vi "Production to internal EEPROM.vi"(8 "error in":errorcluster) -> (0 "error out":errorcluster, 1 "Report":string, 2 "Pass?":bool, 3 "VISA Port":refnum<visa-resource-name>, 5 "DataTime":string, 7 "BOOTVER":string, 10 "BOOTVER":bool, 11 "Time&date":bool)   [LabVIEW 2009]
uses:
  Digit IO PCI 6503/Digit IO control.ctl
  Global/Global 1.vi
  <vilib>/Instr/_visa.llb/VISA Configure Serial Port (Instr).vi
panel:
  out "Path":path=path "E:/LCU6331 test/4821683A000/Config/configration file/Limits_Production.txt"
  out "Interal EEPROM":string
  out "APPVER":bool
  out "APPVER":string
  out "time":timestamp
  out "VerifyTime":string
  out "command Prob2":string
  out "command Prob1":string
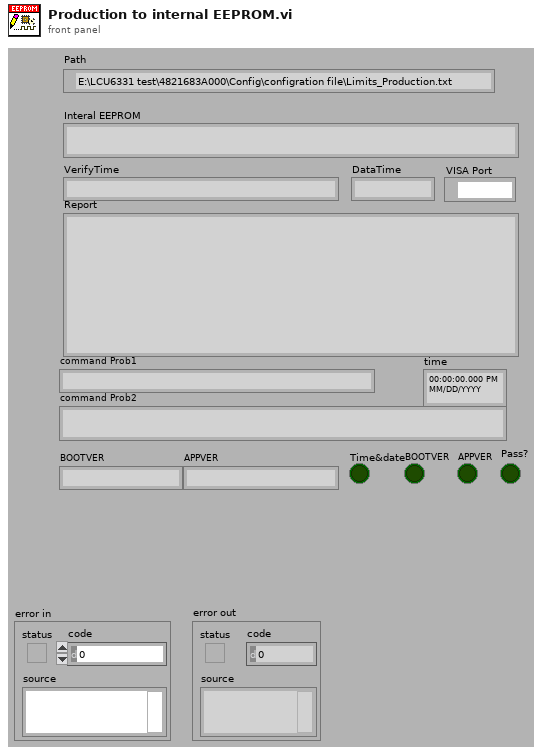
[diagram p1: front panel]
types:
  T1 = typedef "Digit IO control.ctl" = enum16{"Pull X1_4 Low", "Disconnect Pull X1_4 Low", "Down Cylinder", "Disconnect Down Cylinder", "Load X1_1_5", "Disconnect Load X1_1_5", "Measu X1_1_5", "Disconnect Measu X1_1_5", "Measu Z1_1_5", "Disconnect Measu Z1_1_5", "Power X1_1", "Disconnect Power X1_1", "RS232 Power", "Disconnect RS232 Power", "Card Cylinder", "Disconnect Card Cylinder", "Fail LED", "Disconnect Fail LED", "LCA Power", "Disconnect LCA Power", "BeyondCylinderDowndigit", "Disconnect BeyondCylinderDowendigit", "Frequency", "Disconnect Frequency", "Measu Current", "Disconnect Measu Current", "Measu current_1", "Disconnect Measu current_1", "Digit ALL", "Disconnect Digit ALL", "PASS LED", "Disconnect PASS LED", "Load Z1_1_3", "Disconnect Load Z1_1_3", "RS232 Connect", "Disconnect RS232 Connect", "Power Z1_7", "Disconnect Power Z1_7", "Pull Z_1_5  low", "Disconnect Pull Z_1_5  low", "Connect LCA_1", "Disconnect LCA_1", "short LCA", "Disconnect short LCA", "PT100", "Disconnect PT100", "NO connect", "Disconnect NO connect"}
  T2 = enum16{"VHEATFUSENOLOADMIN", "VHEATFUSELOADMAX", "VOVERRIDEDIODEMIN", "TDIFFMAX", "MEASFREQMIN", "MEASFREQMAX", "VMIDDLE", "VUNDER", "VNORESET", "VRESET", "WAITPING", "LRFID", "RFIDUID", "EXTEESIZE", "LCUTYPE", "LCUSUBTYPE", "TEVN", "BOOTVER", "APPVER", "ISLEEPMAX", "TSLEEP", "APPWAIT", "DBWAIT"}[]
  T3 = enum16{"LCU Power on", "Calculating time and date", "Command _E & DATA", "Command_E & String", "Read&Verify data", "Finish"}
  T4 = cluster{"People":string, "product  number":string, "Test time":string, "VHeatFuse_noload":string, "VHeatFuse_load":string, "VoverrideDiode":string, "Test firmware upload via X1":string, "TemperAddress":string, "Troom":string, "TLCU":string, "Adjustment factor":string, "MeasuredFreq":string, "I2C communication":string, "Light-emitting diode on Z2":string, "Battery warning/inhibit":string, "Reset by IC10":string, "External EEPROM":string, "RFID card detection and reading RFID":string, "Production parameters in internal EEPROM":string, "Current consumption in sleep mode":string, "Application and database upload":string, "Test result":string, "Table head[22]":string, "Table head[23]":string}
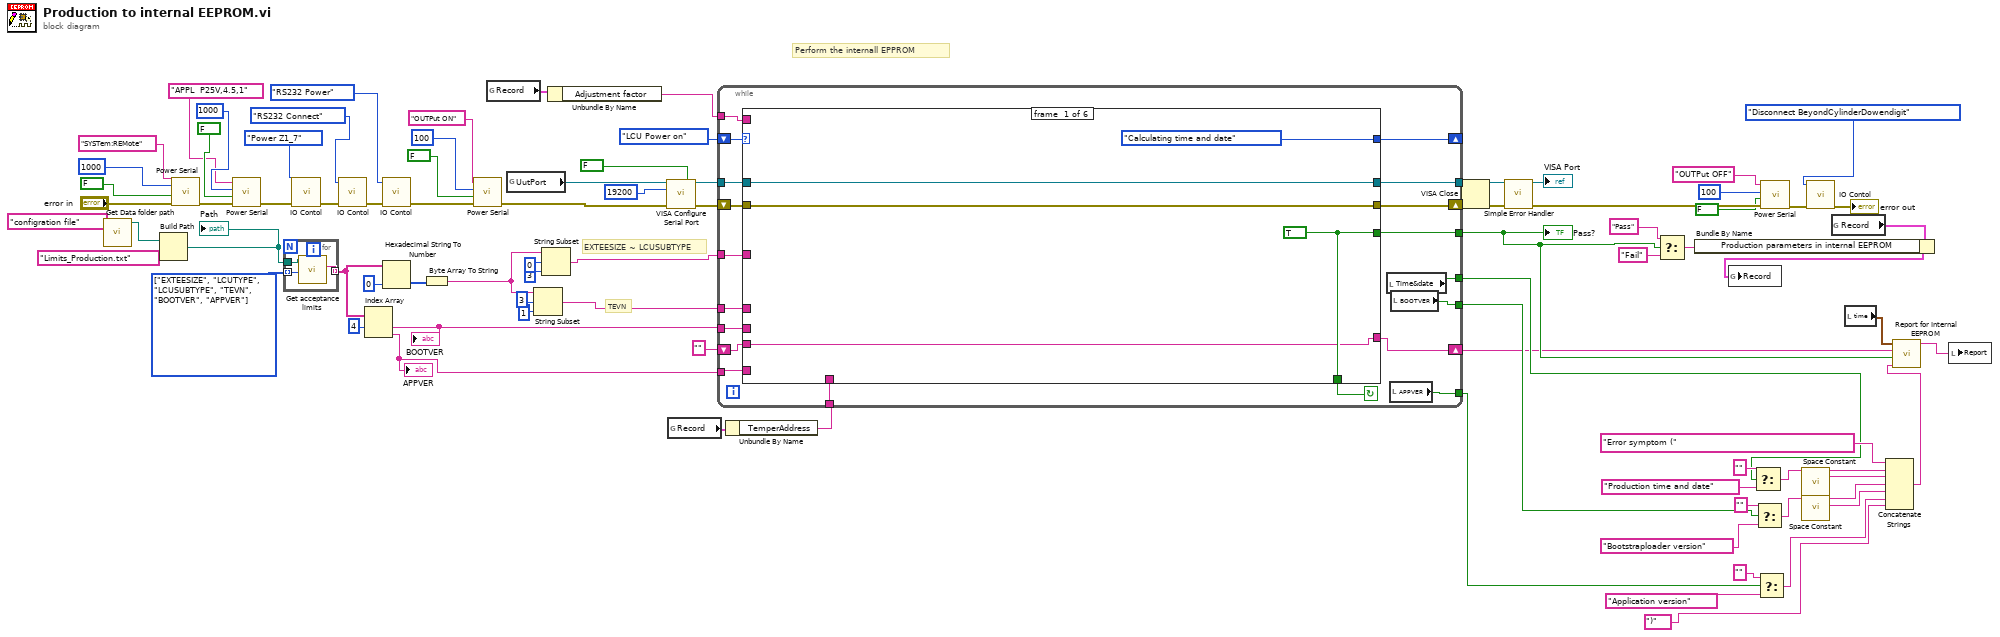
[diagram p0: block diagram]
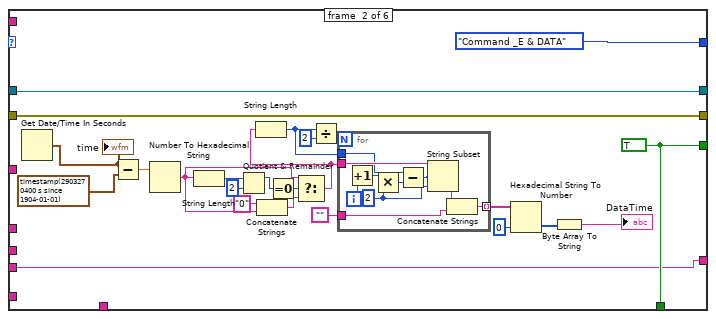
[diagram p2: hidden frame]
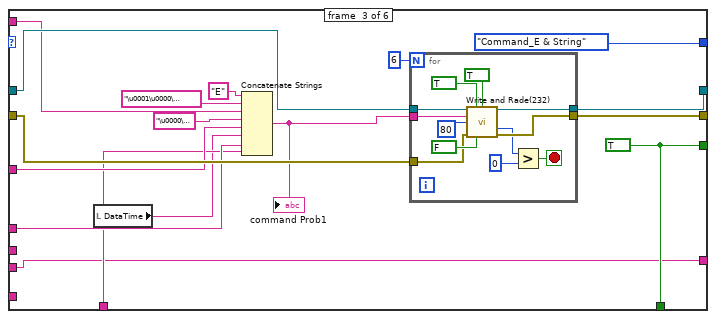
[diagram p3: hidden frame]
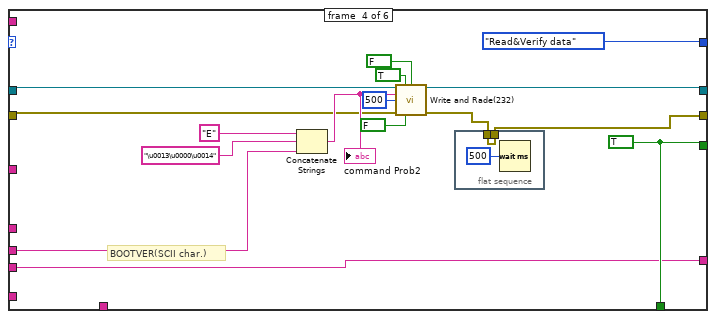
[diagram p4: hidden frame]
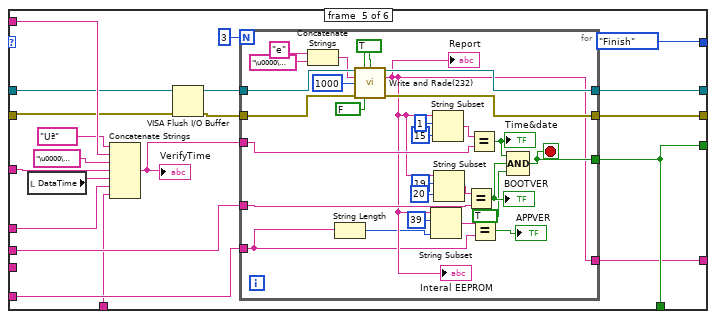
[diagram p5: hidden frame]
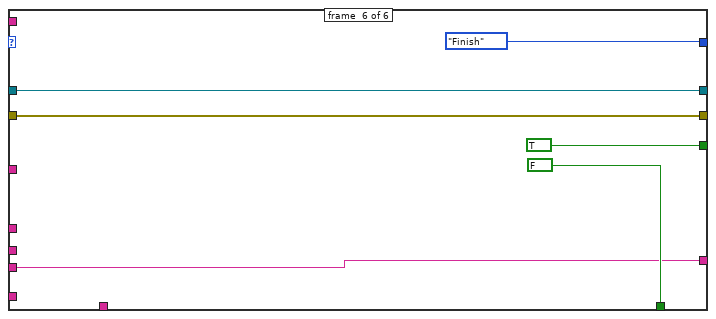
[diagram p6: hidden frame]
diagram:
  w71 = T2 [enum."EXTEESIZE", enum."LCUTYPE", enum."LCUSUBTYPE", enum."TEVN", enum."BOOTVER", enum."APPVER"] items=["VHEATFUSENOLOADMIN", "VHEATFUSELOADMAX", "VOVERRIDEDIODEMIN", "TDIFFMAX", "MEASFREQMIN", "MEASFREQMAX", "VMIDDLE", "VUNDER", "VNORESET", "VRESET", "WAITPING", "LRFID", "RFIDUID", "EXTEESIZE", "LCUTYPE", "LCUSUBTYPE", "TEVN", "BOOTVER", "APPVER", "ISLEEPMAX", "TSLEEP", "APPWAIT", "DBWAIT"]
  # "EXTEESIZE ~ LCUSUBTYPE"
  # "TEVN"
  # "Perform the internall EPPROM"
  n1 = call "Get Data folder path.vi"("Data Path Name"="configration file") -> ("Data Path"=w2:path)  [unwired: 1 in, 9 out]
  n2 = Build Path(base path=w2, name or relative path="Limits_Production.txt") -> (appended path=w1:path)
  "Path" <- w1
  n3 = call "Power Serial.vi"("error in (no error)"="error in", "Rd?"=FALSE, "Delay"=1000, "IN"="SYSTem:REMote" ("In")) -> ("error out"=w53:errorcluster)  [unwired: 1 in, 6 out]
  n4 = call "Power Serial.vi"("error in (no error)"=w53, "Rd?"=FALSE, "Delay"=1000, "IN"="APPL  P25V,4.5,1" ("In")) -> ("error out"=w40:errorcluster)  [unwired: 1 in, 6 out]
  n5 = for {
    tunnel: w1 -> [w87]
    tunnel: [w86] -> w6 mode=indexing
    tunnel: w71 -> [w85] mode=indexing
    n6 = call "Get acceptance limits.vi"("section"=w85, "configuration file path"=w87) -> ("value"=w86:string)  [unwired: 1 in, 8 out]
  }
  n7 = call "IO Contol.vi"("error in"=w40, "IO Operation"=Digit_IO_control."Power Z1_7" ("Enum")) -> ("error out"=w44:errorcluster)  [unwired: 9 out]
  n8 = call "IO Contol.vi"("error in"=w44, "IO Operation"=Digit_IO_control."RS232 Connect" ("Enum")) -> ("error out"=w45:errorcluster)  [unwired: 9 out]
  n9 = Index Array "Index Array"(array=w6, index #1=4 ("index")) -> (element #1=w10:string, element #2=w12:string)  [unwired: 1 in]
  "APPVER" <- w12
  "BOOTVER" <- w10
  n10 = call "IO Contol.vi"("error in"=w45, "IO Operation"=Digit_IO_control."RS232 Power" ("Enum")) -> ("error out"=w36:errorcluster)  [unwired: 9 out]
  n11 = Hexadecimal String To Number(string=w6, default (0uL)=u8 0) -> (number=w5:u8[])  [unwired: 2 out]
  n12 = Byte Array To String(unsigned byte array=w5) -> (string=w66:string)
  n13 = call "Power Serial.vi"("error in (no error)"=w36, "Rd?"=FALSE, "Delay"=100, "IN"="OUTPut ON" ("In")) -> ("error out"=w62:errorcluster)  [unwired: 1 in, 6 out]
  n14 = global read "Global 1.vi" "Record"() -> (w32:T4)
  n15 = global read "Global 1.vi" "UutPort"() -> (w61:refnum<visa-resource-name>)
  n16 = String Subset(string=w66, offset (0)=3, length (rest)=1 ("length (rest)")) -> (substring=w63:string)
  n17 = String Subset(string=w66, offset (0)=0, length (rest)=3 ("length (rest)")) -> (substring=w64:string)
  n18 = Unbundle By Name(w32) -> ("Adjustment factor"=w7:string)
  n19 = call-poly "VISA Configure Serial Port"("VISA resource name"=w61, "Enable Termination\nChar (T)"=FALSE ("Enable Termination\nChar (T)"), "baud rate (9600)"=u32 19200, "error in (no error)"=w62) -> ("VISA resource name out"=w75:refnum<visa-resource-name>, "error out"=w73:errorcluster)  [unwired: 3 in, 7 out]
  n20 = global read "Global 1.vi" "Record"() -> (w60:T4)
  n21 = Unbundle By Name(w60) -> ("TemperAddress"=w59:string)
  n22 = while {
    shift-right: [w99] -> _
    shift-left: T3."LCU Power on" -> [w100]
    tunnel: [w105] -> w76
    tunnel: w75 -> [w104]
    tunnel: [w101] -> w31
    tunnel: w64 -> [w98]
    tunnel: w63 -> [w97]
    tunnel: w10 -> [w96]
    tunnel: w7 -> [w88]
    tunnel: w59 -> [w95]
    shift-right: [w103] -> w74
    shift-left: w73 -> [w102]
    tunnel: [w92] -> w15
    tunnel: [w94] -> w14
    tunnel: w12 -> [w93]
    tunnel: [w91] -> w11
    shift-right: [w90] -> w8
    shift-left: "" ("element") -> [w89]
    stop <- w106 continue-if-true
    n23 = case shown="\"Read&Verify data\"" w100 {
      tunnel: [T3."Calculating time and date" T3."Command _E & DATA" T3."Command_E & String" T3."Read&Verify data" T3."Finish" T3."Finish"] -> w99
      tunnel: [w110 w135 w162 w182 w206 FALSE] -> w106
      tunnel: [w111 w133 w150 w187 w212 w246] -> w105
      tunnel: w104 -> [w111 w133 w161 w188 w194 w246]
      tunnel: [w108 w115 w148 w180 w211 w245] -> w103
      tunnel: w102 -> [w108 w115 w160 w177 w193 w245]
      tunnel: [w110 w135 w162 w182 w206 TRUE] -> w101
      tunnel: w98 -> [_ _ w155 _ w199 _]
      tunnel: w97 -> [_ _ w154 _ w209 _]
      tunnel: w96 -> [_ _ _ w183 w207 _]
      tunnel: w88 -> [_ _ w153 _ w208 _]
      tunnel: w95 -> [_ _ w152 _ w197 _]
      tunnel: w93 -> [_ _ _ _ w203 _]
      tunnel: [w107 w112 w146 w175 w202 w241] -> w90
      tunnel: w89 -> [w107 w112 w146 w175 _ w241]
      frame #0 {
        w110 = TRUE
      }
      frame #1 {
        w135 = TRUE
        n24 = Get Date/Time In Seconds() -> (seconds since 1Jan1904=w113:timestamp)
        "time" <- w113
        n25 = Subtract(x=w113, y=timestamp(2903270400 s since 1904-01-01) ("current time 2")) -> (x-y=w117:dbl)
        n26 = Number To Hexadecimal String(2:w117) -> (0:w132:string)  [unwired: 1 out]
        n27 = String Length(string=w132) -> (length=w120:i32)
        n28 = Quotient & Remainder(x=w120, y=2) -> (x-y*floor(x/y)=w118:i32)  [unwired: 1 out]
        n29 = Concatenate Strings("0" ("string"), w132) -> (w123:string)
        n30 = Equal To 0?(x=w118) -> (x = 0?=w121:bool)
        n31 = Select(t=w132, s=w121, f=w123) -> (s? t:f=w128:string)
        n32 = String Length(string=w128) -> (length=w131:i32)
        n33 = Divide(x=w131, y=2) -> (x/y=w130:dbl)
        n34 = for {
          N: w130 -> [_]
          tunnel: w128 -> [w145]
          tunnel: "" -> [w143]
          tunnel: [w142] -> w127 mode=indexing
          tunnel: w131 -> [w141]
          i -> [w137]
          w138 = 2 ("length (rest)")
          n35 = Increment(x=w137) -> (x+1=w136:i32)
          n36 = Multiply(x=w136, y=w138) -> (x*y=w140:i32)
          n37 = Subtract(x=w141, y=w140) -> (x-y=w139:i32)
          n38 = String Subset(string=w145, offset (0)=w139, length (rest)=w138) -> (substring=w144:string)
          n39 = Concatenate Strings(w144, w143) -> (w142:string)
        }
        n40 = Hexadecimal String To Number(string=w127, default (0uL)=u8 0) -> (number=w126:u8[])  [unwired: 2 out]
        n41 = Byte Array To String(unsigned byte array=w126) -> (string=→"DataTime":string)
      }
      frame #2 {
        w162 = TRUE
        n42 = local read "DataTime"() -> (w149:string)
        n43 = Concatenate Strings("E" ("string to write"), "\u0001\u0000\u000eUª" ("string to write"), w153, "\u0000\u0000" ("string to write"), w155, w149, w154, w152) -> (w151:string)
        "command Prob1" <- w151
        n44 = for {
          N: 6 -> [_]
          tunnel: w161 -> [w172]
          tunnel: w160 -> [w171]
          tunnel: w151 -> [w169]
          tunnel: [w168] -> w150
          tunnel: [w166] -> w148
          stop <- w163 stop-if-true
          n45 = call "Write and Rade(232).vi"("VISA resource name in"=w172, "write"=TRUE, "read"=TRUE, "string to write"=w169, "ms delay"=u32 80 ("millisecond multiple"), "error in"=w171, "change baud rate(read)"=FALSE) -> ("VISA resource name out"=w168:refnum<visa-resource-name>, "bytes read"=w165:u32, "error out"=w166:errorcluster)  [unwired: 1 in, 5 out]
          n46 = Greater?(x=w165, y=u32 0) -> (0:w163:bool)
        }
      }
      frame #3 {
        w182 = TRUE
        # "BOOTVER(SCII char.)"
        n47 = Concatenate Strings("E" ("string to write"), "\u0013\u0000\u0014" ("string to write"), w183) -> (w184:string)
        "command Prob2" <- w184
        n48 = call "Write and Rade(232).vi"("VISA resource name in"=w188, "write"=TRUE, "read"=FALSE, "string to write"=w184, "ms delay"=u32 500 ("millisecond multiple"), "error in"=w177, "change baud rate(read)"=FALSE) -> ("VISA resource name out"=w187:refnum<visa-resource-name>, "error out"=w181:errorcluster)  [unwired: 1 in, 6 out]
        n49 = flat-sequence {
          tunnel: w181 -> [w191]
          tunnel: [w191] -> w180
          frame #0 {
            n50 = Wait (ms)(milliseconds to wait=u32 500) -> ()  [unwired: 1 out]
          }
        }
      }
      frame #4 {
        n51 = local read "DataTime"() -> (w204:string)
        n52 = Concatenate Strings("Uª" ("string to write"), w208, "\u0000\u0000" ("string to write"), w199, w204, w209, w197) -> (w198:string)
        "VerifyTime" <- w198
        n53 = VISA Flush I/O Buffer(VISA resource name=w194, error in (no error)=w193) -> (VISA resource name out=w196:refnum<visa-resource-name>, error out=w195:errorcluster)  [unwired: 1 in]
        n54 = for {
          N: 3 -> [_]
          tunnel: w196 -> [w240]
          tunnel: w195 -> [w239]
          tunnel: [w238] -> w212
          tunnel: [w237] -> w211
          tunnel: w198 -> [w225]
          tunnel: w207 -> [w220]
          tunnel: [w228] -> w206
          tunnel: w203 -> [w215]
          tunnel: [w216] -> w202
          stop <- w228 stop-if-true
          w231 = TRUE ("write")
          n55 = Concatenate Strings("e" ("string to write"), "\u0000\u0000@" ("string to write")) -> (w232:string)
          n56 = String Length(string=w215) -> (length=w214:i32)
          n57 = call "Write and Rade(232).vi"("VISA resource name in"=w240, "write"=w231, "read"=w231, "string to write"=w232, "ms delay"=u32 1000 ("millisecond multiple"), "error in"=w239, "change baud rate(read)"=FALSE) -> ("VISA resource name out"=w238:refnum<visa-resource-name>, "read string"=w216:string, "error out"=w237:errorcluster)  [unwired: 1 in, 5 out]
          "Report" <- w216
          "Interal EEPROM" <- w216
          n58 = String Subset(string=w216, offset (0)=39, length (rest)=w214) -> (substring=w217:string)
          n59 = String Subset(string=w216, offset (0)=1, length (rest)=15 ("length (rest)")) -> (substring=w224:string)
          n60 = String Subset(string=w216, offset (0)=19, length (rest)=20 ("length (rest)")) -> (substring=w219:string)
          n61 = Equal?(x=w219, y=w220) -> (x = y?=w235:bool)
          "BOOTVER" <- w235
          n62 = Equal?(x=w224, y=w225) -> (x = y?=w236:bool)
          "Time&date" <- w236
          n63 = Equal?(x=w217, y=w215) -> (x = y?=→"APPVER":bool)
          n64 = Compound Arithmetic op=AND(w236, w235, TRUE) -> (w228:bool)
        }
      }
      frame #5 {
      }
    }
    n65 = local read "Time&date"() -> (w92:bool)
    n66 = local read "APPVER"() -> (w91:bool)
    n67 = local read "BOOTVER"() -> (w94:bool)
  }
  "VISA Port" <- w76
  "Pass?" <- w31
  n68 = VISA Close(VISA resource name=w76, error in (no error)=w74) -> (error out=w78:errorcluster)
  n69 = call <vilib>:"Simple Error Handler.vi"("error in (no error)"=w78) -> ("error out"=w84:errorcluster)  [unwired: 1 in, 7 out]
  n70 = Select(t="Pass", s=w31, f="Fail") -> (s? t:f=w57:string)
  n71 = Select(t="", s=w15, f="Production time and date") -> (s? t:f=w24:string)
  n72 = Select(t="", s=w14, f="Bootstraploader version") -> (s? t:f=w23:string)
  n73 = Select(t="", s=w11, f="Application version") -> (s? t:f=w17:string)
  n74 = call "Power Serial.vi"("error in (no error)"=w84, "Rd?"=FALSE, "Delay"=100, "IN"="OUTPut OFF" ("In")) -> ("error out"=w83:errorcluster)  [unwired: 1 in, 6 out]
  n75 = call <vilib>:"Space Constant.vi"() -> ("String"=w22:string)
  n76 = call <vilib>:"Space Constant.vi"() -> ("String"=w18:string)
  n77 = call "IO Contol.vi"("error in"=w83, "IO Operation"=Digit_IO_control."Disconnect BeyondCylinderDowendigit") -> ("error out"=→"error out":errorcluster)  [unwired: 9 out]
  n78 = global read "Global 1.vi" "Record"() -> (w58:T4)
  n79 = Bundle By Name(cluster=w58, "Production parameters in internal EEPROM"=w57) -> (w54:T4)
  n80 = global write "Global 1.vi" "Record"(w54) -> ()
  n81 = local read "time"() -> (w30:timestamp)
  n82 = Concatenate Strings("Error symptom (", w24, w22, w23, w18, w17, ")") -> (w13:string)
  n83 = call "Report for Internal EEPROM.vi"("Error"=w13, "Pass?"=w31, "EEPROM contents"=w8, "Time Stamp"=w30) -> ("Report Body"=w29:string)  [unwired: 7 out]
  n84 = local write "Report"(w29) -> ()
